vi "Slow R-T 1.1.vi"() -> ()   [LabVIEW 2024]
uses:
  <vilib>/Utility/file.llb/Write Delimited Spreadsheet (DBL).vi
panel:
  in  "stop":bool
  in  "Tab Control 2":enum32{"cRIO", "Lockin X", "Lockin Y"}(tab)
  out "cRIO":cluster{"Y":dbl[], "Y":dbl[]}[](graph)
  out "Chan0":string="DC Voltage V"
  out "Chan1":string="DC current uA"
  out "Chan2":string="dV V"
  out "Chan 4":string="dI uA"
  out "Lockin X":cluster{"Y":dbl[], "Y":dbl[]}[](graph)
  out "Lockin Y":cluster{"Y":dbl[], "Y":dbl[]}[](graph)
  in  "Tab Control":enum32{"cRIO", "Temp", "Lockin", "Status"}(tab)
  in  "Chan 0":bool=TRUE
  in  "cRIO IP":string="//172.22.11.2"
  in  "Reading Average times":i32=20
  in  "AO Channel":string(combo)="AO0"
  in  "Current output Scale factor":dbl=10.0
  in  "Current Start uA":dbl=0.5
  in  "Scale factor0":dbl=0.0001
  in  "Channel name 0":string(combo)="DC Voltage V"
  in  "Channel name 1":string(combo)="DC current uA"
  in  "Chan 1":bool=TRUE
  in  "Scale factor1":dbl=2.0
  in  "Channel name 2":string(combo)="dV V"
  in  "Chan 2":bool
  in  "Scale factor2":dbl=1.0
  in  "Channel name 3":string(combo)="dI uA"
  in  "Chan 3":bool
  in  "Scale factor3":dbl=1.0
  in  "Delay Time s":dbl=30.0 caption="Delay Time (s)"
  in  "Device":string(combo)="Elsa"
  in  "Temp Chan":string="T5"
  in  "Lockin address 4":string
  in  "Lockin address 3":string
  in  "Lockin address 2":string="GPIB0::9::INSTR"
  in  "Lockin address 1":string="GPIB0::8::INSTR"
  in  "Lockin 4":bool
  in  "Lockin 3":bool
  in  "Lockin 2":bool
  in  "Lockin 1":bool
  in  "Use Lockin":bool
  in  "Lockin Chan name 4":string(combo)="None"
  in  "Lockin Chan name 3":string(combo)="None"
  in  "Lockin Chan name 2":string(combo)="mV"
  in  "Lockin Chan name 1":string(combo)="mV"
  in  "Status":string="Data File time stamp 20210306-203251\nmagnetic field -4.996000mT\nLockin status\n"
  in  "Magnetic field read device":string(combo)="Elsa Magnet"
  in  "Record Field":bool=TRUE
  in  "Contour plot folder":path=path "C:/Users/sureshb2/Desktop/Measurements/3782"
  out "error out":errorcluster
  # "Voltage x factor=uA"
  # "Voltage x factor=actual"
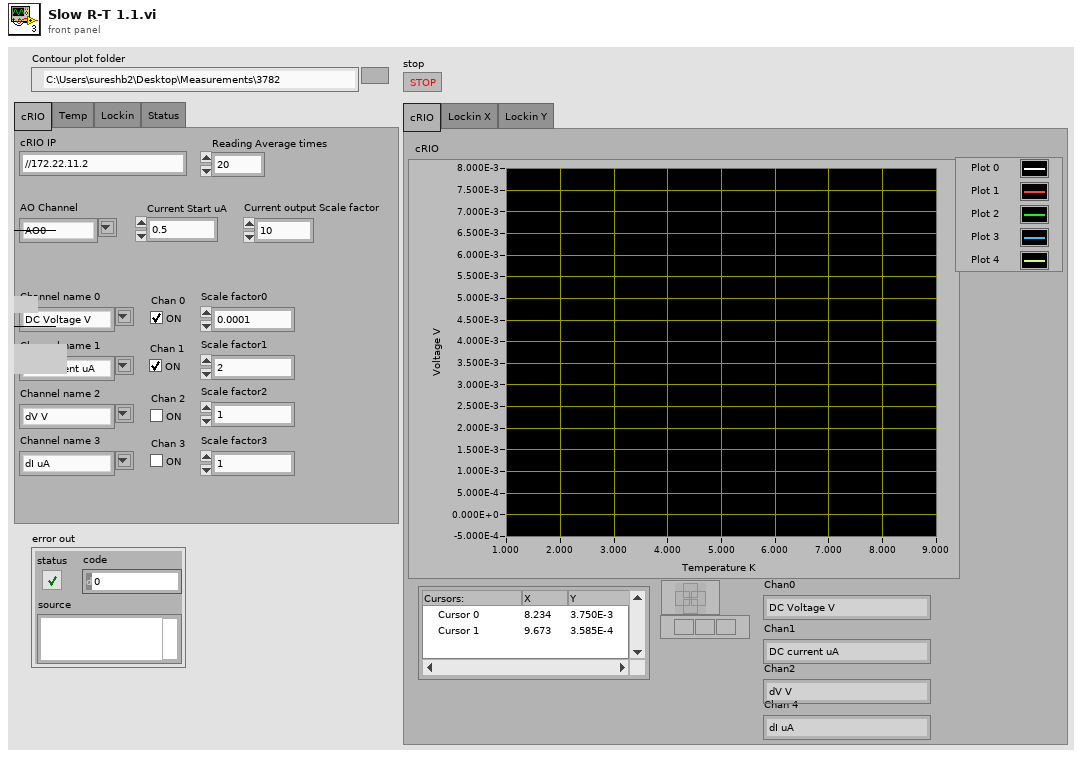
[diagram p1: front panel]
types:
  T1 = cluster{"AI0":dbl, "AI1":dbl, "AI2":dbl, "AI3":dbl}
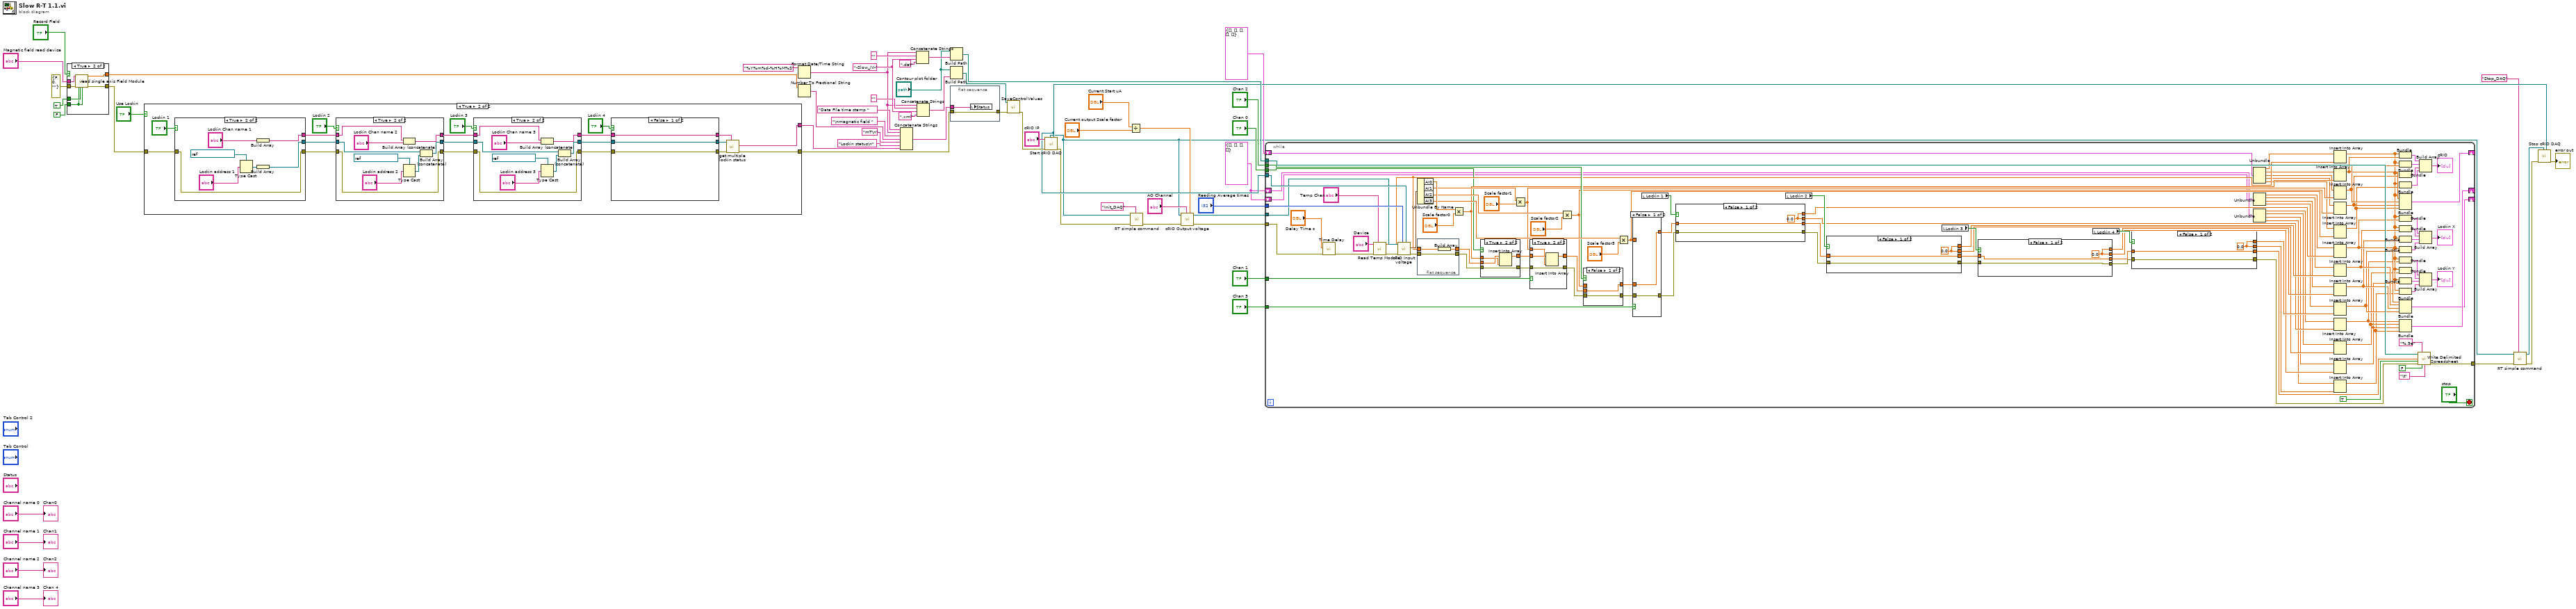
[diagram p0: block diagram]
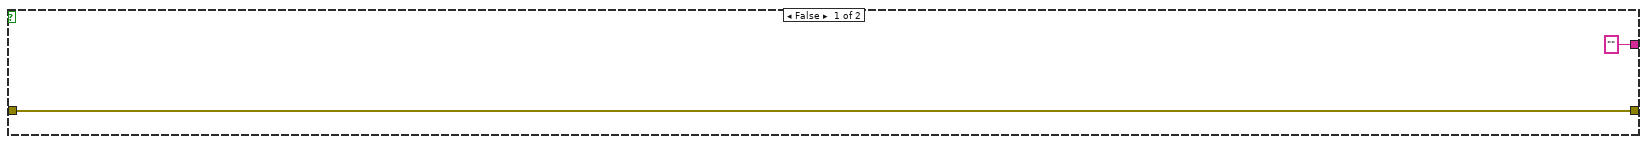
[diagram p2: hidden frame]
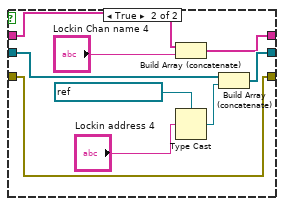
[diagram p3: hidden frame]
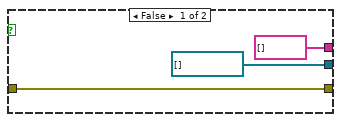
[diagram p6: hidden frame]
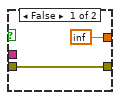
[diagram p7: hidden frame]
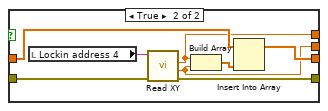
[diagram p8: hidden frame]
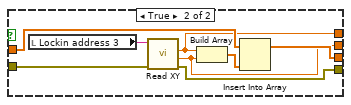
[diagram p9: hidden frame]
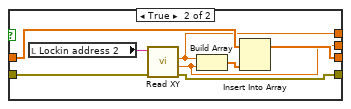
[diagram p10: hidden frame]
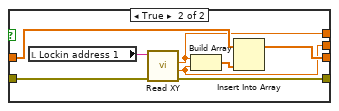
[diagram p11: hidden frame]
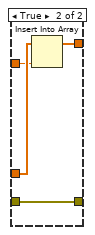
[diagram p13: hidden frame]
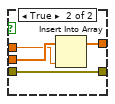
[diagram p14: hidden frame]
diagram:
  w9 = cluster{dbl[], dbl[], dbl[], dbl[]} {[], [], [], []} ("output cluster")
  w52 = "-Slow_IV-"
  n1 = case shown="True" "Record Field" {
    tunnel: errorcluster {"status"=FALSE, "code"=0, "source"=""} ("error in") -> [w60 w66]
    tunnel: "Magnetic field read device" -> [_ w65]
    tunnel: [inf w64] -> w16
    tunnel: TRUE ("Exec") -> [_ w63]
    tunnel: FALSE ("Init") -> [_ w62]
    tunnel: [w60 w61] -> w23
    frame False {
    }
    frame True {
      n2 = call "read single axis Field Module.vi"("Magnet Device Select"=w65, "error in (no error)"=w66, "Init"=w62, "Exec"=w63, "final"=w62) -> ("FIeld mT"=w64:dbl, "error out"=w61:errorcluster)  [unwired: 13 in]
    }
  }
  n3 = case shown="True" "Use Lockin" {
    tunnel: ["" ("Status output") w87] -> w15
    tunnel: [w68 w86] -> w13
    tunnel: w23 -> [w68 w85]
    frame False {
    }
    frame True {
      n4 = case shown="True" "Lockin 1" {
        tunnel: w85 -> [w125 w133]
        tunnel: [w125 w133] -> w84
        tunnel: [refnum<visa-resource-name>[] [] w132] -> w80
        tunnel: [string[] [] w131] -> w76
        frame False {
        }
        frame True {
          n5 = Type Cast(type=refnum<visa-resource-name> "GPIB0::8::INSTR" ("Lockin address 1"), x="Lockin address 1") -> (*(type *) &x=w129:refnum<visa-resource-name>)
          n6 = Build Array("Lockin Chan name 1") -> (w131:string[])
          n7 = Build Array(w129) -> (w132:refnum<visa-resource-name>[])
        }
      }
      n8 = case shown="True" "Lockin 2" {
        tunnel: w84 -> [w113 w123]
        tunnel: [w113 w123] -> w83
        tunnel: w80 -> [w114 w122]
        tunnel: [w114 w121] -> w79
        tunnel: w76 -> [w112 w120]
        tunnel: [w112 w119] -> w75
        frame False {
        }
        frame True {
          n9 = Build Array (concatenate)(w120, "Lockin Chan name 2") -> (w119:string[])
          n10 = Type Cast(type=refnum<visa-resource-name> "GPIB0::8::INSTR" ("Lockin address 1"), x="Lockin address 2") -> (*(type *) &x=w117:refnum<visa-resource-name>)
          n11 = Build Array (concatenate)(w122, w117) -> (w121:refnum<visa-resource-name>[])
        }
      }
      n12 = case shown="True" "Lockin 3" {
        tunnel: w83 -> [w101 w111]
        tunnel: [w101 w111] -> w82
        tunnel: w79 -> [w102 w110]
        tunnel: [w102 w109] -> w78
        tunnel: w75 -> [w100 w108]
        tunnel: [w100 w107] -> w74
        frame False {
        }
        frame True {
          n13 = Build Array (concatenate)(w108, "Lockin Chan name 3") -> (w107:string[])
          n14 = Type Cast(type=refnum<visa-resource-name> "GPIB0::8::INSTR" ("Lockin address 1"), x="Lockin address 3") -> (*(type *) &x=w105:refnum<visa-resource-name>)
          n15 = Build Array (concatenate)(w110, w105) -> (w109:refnum<visa-resource-name>[])
        }
      }
      n16 = case shown="False" "Lockin 4" {
        tunnel: w82 -> [w89 w99]
        tunnel: [w89 w99] -> w81
        tunnel: w78 -> [w90 w98]
        tunnel: [w90 w97] -> w77
        tunnel: w74 -> [w88 w93]
        tunnel: [w88 w92] -> w69
        frame False {
        }
        frame True {
          n17 = Build Array (concatenate)(w93, "Lockin Chan name 4") -> (w92:string[])
          n18 = Type Cast(type=refnum<visa-resource-name> "GPIB0::8::INSTR" ("Lockin address 1"), x="Lockin address 4") -> (*(type *) &x=w95:refnum<visa-resource-name>)
          n19 = Build Array (concatenate)(w98, w95) -> (w97:refnum<visa-resource-name>[])
        }
      }
      n20 = call "get multiple lockin status.vi"("Device channel names"=w69, "error in (no error)"=w81, "SRS830 addresses"=w77) -> ("error out"=w86:errorcluster, "Status output"=w87:string)  [unwired: 6 in, 1 out]
    }
  }
  n21 = Format Date/Time String(time format string (%c)="%Y%m%d-%H%M%S") -> (date/time string=w17:string)  [unwired: 2 in]
  n22 = Number To Fractional String(number=w16) -> (F-format string=w20:string)  [unwired: 3 in]
  n23 = Concatenate Strings("Data File time stamp " ("string"), w17, "\nmagnetic field " ("string"), w20, "mT\n" ("string"), "Lockin status\n" ("string"), w15) -> (w14:string)
  n24 = Concatenate Strings(w17, "" ("string"), w52, ".dat" ("string")) -> (w54:string)
  n25 = Concatenate Strings(w17, "" ("string"), w52, ".xml" ("string")) -> (w57:string)
  n26 = Build Path(base path="Contour plot folder", name or relative path=w54) -> (appended path=w46:path)
  n27 = Build Path(base path="Contour plot folder", name or relative path=w57) -> (appended path=w55:path)
  n28 = flat-sequence {
    tunnel: w14 -> [w135]
    tunnel: w13 -> [w134]
    tunnel: [w134] -> w12
    frame #0 {
      n29 = local write "Status"(w135) -> ()
    }
  }
  n30 = call "SaveControlValues.vi"("XML File Path"=w55, "error in (no error)"=w12) -> ("error out"=w50:errorcluster)  [unwired: 8 in]
  n31 = call "Start cRIO DAQ.vi"("error in (no error)"=w50, "cRIO IP"="cRIO IP") -> ("error out"=w7:errorcluster, "DAQ_AI_Reader endpoint"=w45:refnum<k21>, "DAQ_CMD_Writer endpoint"=w4:refnum<k21>)  [unwired: 7 in]
  n32 = Divide(x="Current Start uA", y="Current output Scale factor") -> (x/y=w32:dbl)
  n33 = call "RT simple command.vi"("Command"="Init_DAQ", "error in (no error)"=w7, "DAQ_CMD_Writer endpoint"=w4) -> ("error out"=w6:errorcluster)  [unwired: 7 in, 1 out]
  n34 = call "cRIO Output voltage.vi"("Voltage"=w32, "AO Channel"="AO Channel", "error in (no error)"=w6, "DAQ_CMD_Writer endpoint"=w4) -> ("error out"=w31:errorcluster, "DAQ_CMD_Writer endpoint out"=w30:refnum<k21>)  [unwired: 6 in]
  n35 = while {
    tunnel: w31 -> [w247]
    tunnel: w45 -> [w246]
    tunnel: w46 -> [w245]
    tunnel: "Chan 1" -> [w231]
    tunnel: "Chan 2" -> [w230]
    tunnel: "Chan 3" -> [w229]
    tunnel: [w223] -> w3
    tunnel: "Reading Average times" -> [w219]
    tunnel: w30 -> [w217]
    tunnel: "Chan 0" -> [w205]
    shift-right: [w204] -> _
    shift-left: cluster{dbl[], dbl[], dbl[], dbl[], dbl[]} {[], [], [], [], []} ("output cluster") -> [w203]
    shift-right: [w166] -> _
    shift-left: w9 -> [w144]
    shift-right: [w165] -> _
    shift-left: w9 -> [w145]
    stop <- "stop" stop-if-true
    n36 = call "Time Delay"("error in (no error)"=w247, "Delay Time (s)"="Delay Time s") -> ("error out"=w216:errorcluster)  [unwired: 9 in]
    n37 = call "Read Temp Module.vi"("Temp Chan"="Temp Chan", "error in (no error)"=w216, "Device"="Device") -> ("error out"=w215:errorcluster, "Temperature K"=w214:dbl)  [unwired: 7 in]
    n38 = call "cRIO Input voltage.vi"("DAQ_AI_Reader endpoint"=w246, "Average"=w219, "error in (no error)"=w215, "DAQ_CMD_Writer endpoint"=w217) -> ("error out"=w226:errorcluster, "output cluster"=w241:T1)  [unwired: 5 in, 1 out]
    n39 = Unbundle By Name(w241) -> ("AI0"=w240:dbl, "AI1"=w239:dbl, "AI2"=w238:dbl, "AI3"=w237:dbl)
    n40 = flat-sequence {
      tunnel: w226 -> [w300]
      tunnel: [w300] -> w210
      tunnel: [w299] -> w208
      tunnel: w214 -> [w298]
      frame #0 {
        n41 = Build Array(w298) -> (w299:dbl[])
      }
    }
    n42 = Multiply(x=w240, y="Scale factor0") -> (x*y=w207:dbl)
    n43 = case shown="True" w205 {
      tunnel: w210 -> [w292 w297]
      tunnel: [w292 w297] -> w209
      tunnel: w208 -> [w293 w296]
      tunnel: w207 -> [_ w295]
      tunnel: [w293 w294] -> w206
      frame False {
      }
      frame True {
        n44 = Insert Into Array(array=w296, new element=w295) -> (w294:dbl[])  [unwired: 1 in]
      }
    }
    n45 = Multiply(x=w239, y="Scale factor1") -> (x*y=w222:dbl)
    n46 = case shown="True" w231 {
      tunnel: w209 -> [w313 w318]
      tunnel: [w313 w318] -> w228
      tunnel: w206 -> [w314 w317]
      tunnel: w222 -> [_ w316]
      tunnel: [w314 w315] -> w225
      frame False {
      }
      frame True {
        n47 = Insert Into Array(array=w317, new element=w316) -> (w315:dbl[])  [unwired: 1 in]
      }
    }
    n48 = Multiply(x=w238, y="Scale factor2") -> (x*y=w221:dbl)
    n49 = case shown="False" w230 {
      tunnel: w228 -> [w307 w312]
      tunnel: [w307 w312] -> w227
      tunnel: w225 -> [w308 w311]
      tunnel: w221 -> [_ w310]
      tunnel: [w308 w309] -> w224
      frame False {
      }
      frame True {
        n50 = Insert Into Array(array=w311, new element=w310) -> (w309:dbl[])  [unwired: 1 in]
      }
    }
    n51 = Multiply(x=w237, y="Scale factor3") -> (x*y=w220:dbl)
    n52 = case shown="False" w229 {
      tunnel: w227 -> [w301 w303]
      tunnel: w224 -> [w302 w306]
      tunnel: w220 -> [_ w305]
      tunnel: [w302 w304] -> w179
      tunnel: [w301 w303] -> w188
      frame False {
      }
      frame True {
        n53 = Insert Into Array(array=w306, new element=w305) -> (w304:dbl[])  [unwired: 1 in]
      }
    }
    n54 = local read "Lockin 1"() -> (w183:bool)
    n55 = case shown="False" w183 {
      tunnel: w188 -> [w282 w289]
      tunnel: w179 -> [w283 w286]
      tunnel: [w283 w287] -> w178
      tunnel: [w282 w288] -> w187
      tunnel: [w281 w285] -> w174
      tunnel: [w281 w284] -> w170
      frame False {
        w281 = 0.0 ("X mV")
      }
      frame True {
        n56 = local read "Lockin address 1"() -> (w290:string)
        n57 = call "Read XY.vi"("error in (no error)"=w289, "VISA resource name"=w290) -> ("error out"=w288:errorcluster, "Y mV"=w284:dbl, "X mV"=w285:dbl)  [unwired: 5 in, 2 out]
        n58 = Build Array(w285, w284) -> (w291:dbl[])
        n59 = Insert Into Array(array=w286, new element=w291) -> (w287:dbl[])  [unwired: 1 in]
      }
    }
    n60 = local read "Lockin 2"() -> (w182:bool)
    n61 = case shown="False" w182 {
      tunnel: w187 -> [w271 w278]
      tunnel: w178 -> [w272 w275]
      tunnel: [w272 w276] -> w177
      tunnel: [w271 w277] -> w186
      tunnel: [w270 w274] -> w173
      tunnel: [w270 w273] -> w169
      frame False {
        w270 = 0.0 ("X mV")
      }
      frame True {
        n62 = local read "Lockin address 2"() -> (w279:string)
        n63 = call "Read XY.vi"("error in (no error)"=w278, "VISA resource name"=w279) -> ("error out"=w277:errorcluster, "Y mV"=w273:dbl, "X mV"=w274:dbl)  [unwired: 5 in, 2 out]
        n64 = Build Array(w274, w273) -> (w280:dbl[])
        n65 = Insert Into Array(array=w275, new element=w280) -> (w276:dbl[])  [unwired: 1 in]
      }
    }
    n66 = local read "Lockin 3"() -> (w181:bool)
    n67 = case shown="False" w181 {
      tunnel: w186 -> [w260 w267]
      tunnel: w177 -> [w261 w264]
      tunnel: [w261 w265] -> w176
      tunnel: [w260 w266] -> w185
      tunnel: [w259 w263] -> w172
      tunnel: [w259 w262] -> w168
      frame False {
        w259 = 0.0 ("X mV")
      }
      frame True {
        n68 = local read "Lockin address 3"() -> (w268:string)
        n69 = call "Read XY.vi"("error in (no error)"=w267, "VISA resource name"=w268) -> ("error out"=w266:errorcluster, "Y mV"=w262:dbl, "X mV"=w263:dbl)  [unwired: 5 in, 2 out]
        n70 = Build Array(w263, w262) -> (w269:dbl[])
        n71 = Insert Into Array(array=w264, new element=w269) -> (w265:dbl[])  [unwired: 1 in]
      }
    }
    n72 = local read "Lockin 4"() -> (w180:bool)
    n73 = case shown="False" w180 {
      tunnel: w185 -> [w249 w256]
      tunnel: w176 -> [w250 w253]
      tunnel: [w250 w254] -> w175
      tunnel: [w249 w255] -> w184
      tunnel: [w248 w252] -> w171
      tunnel: [w248 w251] -> w167
      frame False {
        w248 = 0.0 ("X mV")
      }
      frame True {
        n74 = local read "Lockin address 4"() -> (w257:string)
        n75 = call "Read XY.vi"("error in (no error)"=w256, "VISA resource name"=w257) -> ("error out"=w255:errorcluster, "Y mV"=w251:dbl, "X mV"=w252:dbl)  [unwired: 5 in, 2 out]
        n76 = Build Array(w252, w251) -> (w258:dbl[])
        n77 = Insert Into Array(array=w253, new element=w258) -> (w254:dbl[])  [unwired: 1 in]
      }
    }
    n78 = Unbundle(w203) -> (w202:dbl[], w201:dbl[], w200:dbl[], w199:dbl[], w198:dbl[])
    n79 = Unbundle(w145) -> (w143:dbl[], w142:dbl[], w141:dbl[], w140:dbl[])
    n80 = Unbundle(w144) -> (w139:dbl[], w138:dbl[], w137:dbl[], w136:dbl[])
    n81 = Insert Into Array(array=w202, new element=w214) -> (w150:dbl[])  [unwired: 1 in]
    n82 = Insert Into Array(array=w201, new element=w207) -> (w197:dbl[])  [unwired: 1 in]
    n83 = Insert Into Array(array=w200, new element=w222) -> (w196:dbl[])  [unwired: 1 in]
    n84 = Insert Into Array(array=w199, new element=w221) -> (w195:dbl[])  [unwired: 1 in]
    n85 = Insert Into Array(array=w198, new element=w220) -> (w194:dbl[])  [unwired: 1 in]
    n86 = Insert Into Array(array=w143, new element=w174) -> (w156:dbl[])  [unwired: 1 in]
    n87 = Insert Into Array(array=w142, new element=w173) -> (w155:dbl[])  [unwired: 1 in]
    n88 = Insert Into Array(array=w141, new element=w172) -> (w154:dbl[])  [unwired: 1 in]
    n89 = Insert Into Array(array=w140, new element=w171) -> (w153:dbl[])  [unwired: 1 in]
    n90 = Insert Into Array(array=w139, new element=w170) -> (w149:dbl[])  [unwired: 1 in]
    n91 = Insert Into Array(array=w138, new element=w169) -> (w148:dbl[])  [unwired: 1 in]
    n92 = Insert Into Array(array=w137, new element=w168) -> (w147:dbl[])  [unwired: 1 in]
    n93 = Insert Into Array(array=w136, new element=w167) -> (w146:dbl[])  [unwired: 1 in]
    n94 = Bundle(w150, w197) -> (w193:cluster{dbl[], dbl[]})  [unwired: 1 in]
    n95 = Bundle(w150, w196) -> (w192:cluster{dbl[], dbl[]})  [unwired: 1 in]
    n96 = Bundle(w150, w195) -> (w191:cluster{dbl[], dbl[]})  [unwired: 1 in]
    n97 = Bundle(w150, w194) -> (w190:cluster{dbl[], dbl[]})  [unwired: 1 in]
    n98 = Bundle(w150, w197, w196, w195, w194) -> (w204:cluster{dbl[], dbl[], dbl[], dbl[], dbl[]})  [unwired: 1 in]
    n99 = Bundle(w150, w156) -> (w164:cluster{dbl[], dbl[]})  [unwired: 1 in]
    n100 = Bundle(w150, w155) -> (w163:cluster{dbl[], dbl[]})  [unwired: 1 in]
    n101 = Bundle(w150, w154) -> (w162:cluster{dbl[], dbl[]})  [unwired: 1 in]
    n102 = Bundle(w150, w153) -> (w161:cluster{dbl[], dbl[]})  [unwired: 1 in]
    n103 = Bundle(w150, w149) -> (w160:cluster{dbl[], dbl[]})  [unwired: 1 in]
    n104 = Bundle(w150, w148) -> (w159:cluster{dbl[], dbl[]})  [unwired: 1 in]
    n105 = Bundle(w150, w147) -> (w158:cluster{dbl[], dbl[]})  [unwired: 1 in]
    n106 = Bundle(w150, w146) -> (w157:cluster{dbl[], dbl[]})  [unwired: 1 in]
    n107 = Bundle(w156, w155, w154, w153) -> (w165:cluster{dbl[], dbl[], dbl[], dbl[]})  [unwired: 1 in]
    n108 = Bundle(w149, w148, w147, w146) -> (w166:cluster{dbl[], dbl[], dbl[], dbl[]})  [unwired: 1 in]
    n109 = call-poly <vilib>:"Write Delimited Spreadsheet.vi"("file path (dialog if empty)"=w245, "format (%.3f)"="%.9e", "1D data"=w175, "append to file? (new file:F)"=TRUE, "error in (no error)"=w184, "transpose? (no:F)"=FALSE, "delimiter (\\t)"="\t" ("delimiter (\\t)")) -> ("error out"=w223:errorcluster)  [unwired: 7 in, 1 out]
    n110 = Build Array(w193, w192, w191, w190) -> (→"cRIO":cluster{dbl[], dbl[]}[])
    n111 = Build Array(w164, w163, w162, w161) -> (→"Lockin X":cluster{dbl[], dbl[]}[])
    n112 = Build Array(w160, w159, w158, w157) -> (→"Lockin Y":cluster{dbl[], dbl[]}[])
  }
  n113 = call "RT simple command.vi"("Command"="Stop_DAQ", "error in (no error)"=w3, "DAQ_CMD_Writer endpoint"=w4) -> ("error out"=w2:errorcluster, "DAQ_CMD_Writer endpoint out"=w5:refnum<k21>)  [unwired: 7 in]
  n114 = call "Stop cRIO DAQ.vi"("DAQ_AI_Reader endpoint"=w45, "DAQ_CMD_Writer endpoint"=w5, "error in (no error)"=w2) -> ("error out"=→"error out":errorcluster)  [unwired: 8 in]
  "Chan0" <- "Channel name 0"
  "Chan1" <- "Channel name 1"
  "Chan2" <- "Channel name 2"
  "Chan 4" <- "Channel name 3"
